vi "WristGlobal.vi"() -> ()   [LabVIEW 2023]
panel:
  out "WristProtectLowLimitClampActive":bool
  out "WristProtectHighLimitClampActive":bool
  out "WristBeforeClampSetpoint":dbl
  out "WristMotorGravityComp":dbl
  in  "WristAtSetpoint":bool
  out "WristAbsSensor":dbl
  out "WristMotorOutput":dbl
  in  "CurrentWristSetpoint":dbl
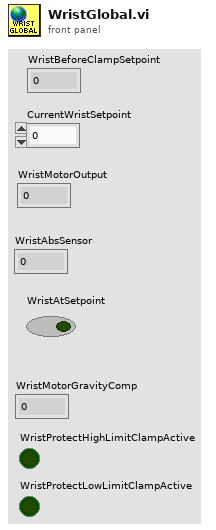
[diagram p1: front panel]
diagram:
